vi "G# - InterfaceDemo2.vi"() -> ()   [LabVIEW 2017]
doc: "G# Interface Implementation\nThis examples demonstrates how to use the G#Interface. The interface concept is an alternative design principle to multiple inheritance (just as in C# and Java). Classes that are not related can implement the same interface and the reference of the interface could be treated just as they are from the same class.\n\nBy using the G# Debugger found in Tools->G# Debugger a text log can be followed showing how the objects were created and destroyed."
uses:
  IMyInterface2_interface/IMyInterface2.lvclass
  C:/ProjectGSharpDevelopment_2017/gsharp/VIPM/Files/vi.lib/addons/_AddQ/G#Object/G#Object.lvclass
  MyClass3_class/MyClass3.lvclass
  MyClass4_class/MyClass4.lvclass
  vi.lib/addons/_AddQ/G#Object/G#Object.lvclass
panel:
  out "# of objects killed":i32
  out "OK":bool
  in  "error in (no error)":errorcluster
  out "MyClass4 is instance of IMyInterface":bool
  out "MyClass3 is instance of IMyInterface":bool
  out "error out":errorcluster
  out "Class Name":string[](array[string])
  # "G# Interface Implementation without wrapper classes\nThis examples demonstrates how to use the G#Interface without using wrapper classes. The interface concept is an alternative design principle to multiple inheritance (just as in C# and Java).\nClasses that are not related can implement the same interface and the reference of the interface could be treated just as they are from the same class.\n\nBy using the G# Debugger found in Tools->G# Debugger a text log can be followed showing how the objects were created and destroyed."
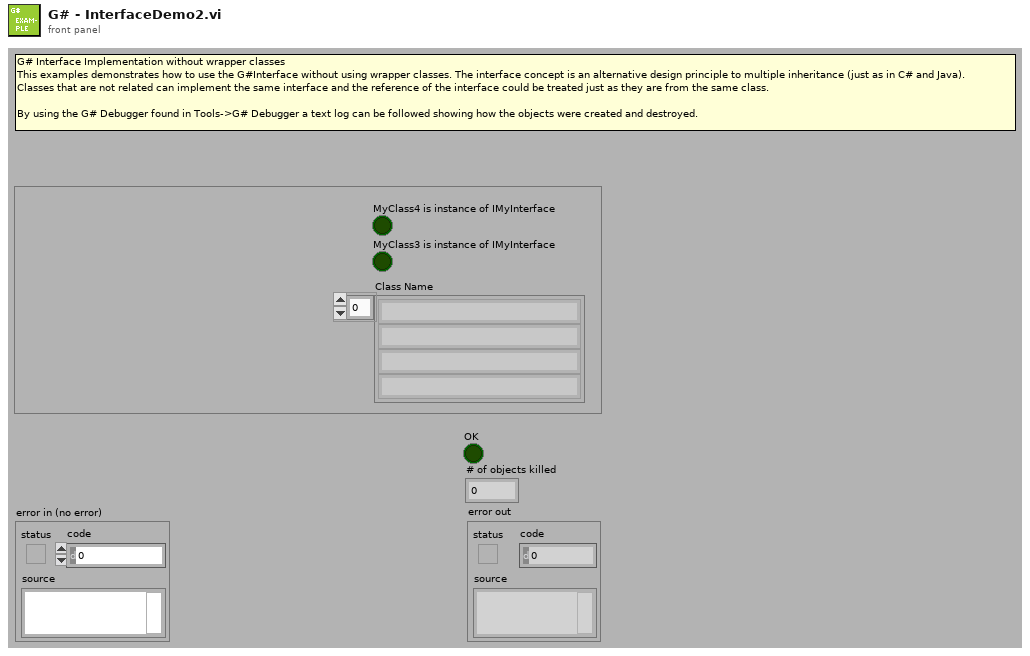
[diagram p1: front panel]
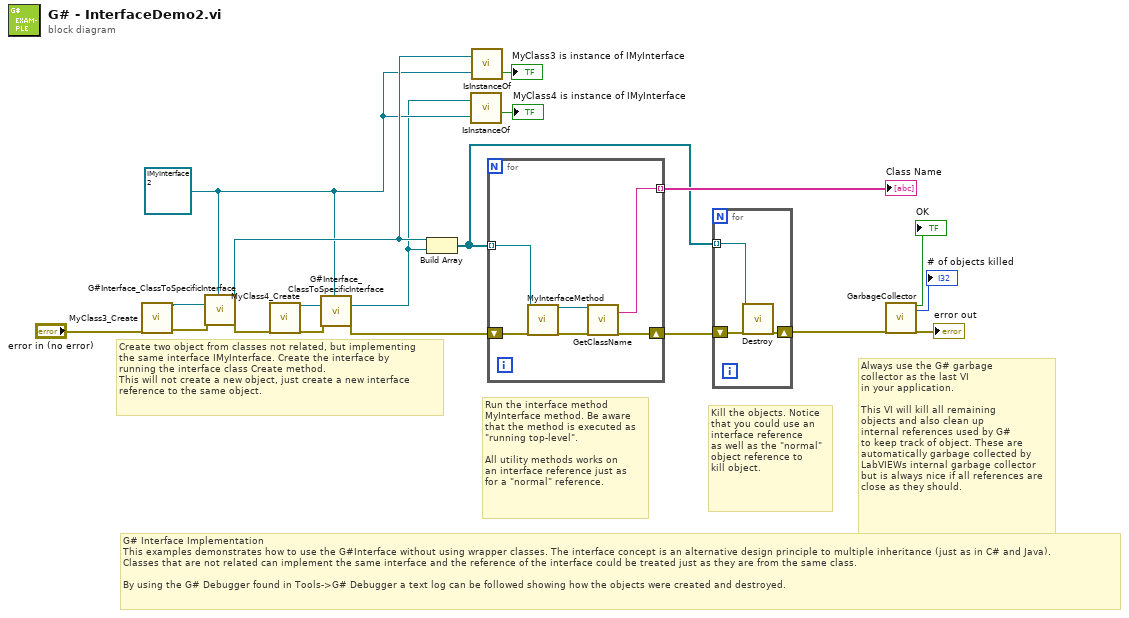
[diagram p0: block diagram]
diagram:
  w2 = refnum<class "IMyInterface2.lvclass"> refnum ("IMyInterface2.lvclass")
  # "G# Interface Implementation\nThis examples demonstrates how to use the G#Interface without using wrapper classes. The interface concept is an alternative design principle to multiple inheritance (just as in C# and Java).\nClasses that are not related can implement the same interface and the reference of the interface could be treated just as they are from the same class.\n\nBy using the G# Debugger found in Tools->G# Debugger a text log can be followed showing how the objects were created and destroyed."
  # "Always use the G# garbage\ncollector as the last VI\nin your application.\n\nThis VI will kill all remaining\nobjects and also clean up\ninternal references used by G#\nto keep track of object. These are\nautomatically garbage collected by\nLabVIEWs internal garbage collector\nbut is always nice if all references are\nclose as they should."
  # "Kill the objects. Notice\nthat you could use an\ninterface reference\nas well as the \"normal\"\nobject reference to\nkill object."
  # "Run the interface method\nMyInterface method. Be aware\nthat the method is executed as\n\"running top-level\".\n\nAll utility methods works on\nan interface reference just as\nfor a \"normal\" reference."
  # "Create two object from classes not related, but implementing\nthe same interface IMyInterface. Create the interface by\nrunning the interface class Create method.\nThis will not create a new object, just create a new interface\nreference to the same object."
  n1 = call "MyClass3_Create.vi"("error in (no error)"="error in (no error)") -> ("reference out"=w7:refnum<class "MyClass3.lvclass">, "error out"=w9:errorcluster)  [unwired: 17 in]
  n2 = call-dynamic "G#Interface_ClassToSpecificInterface.vi"("reference in"=w7, "error in (no error)"=w9, "target interface"=w2) -> ("interface reference out"=w6:refnum<class "IMyInterface2.lvclass">, "error out"=w8:errorcluster)  [unwired: 23 in]
  n3 = call "MyClass4_Create.vi"("error in (no error)"=w8) -> ("reference out"=w5:refnum<class "MyClass4.lvclass">, "error out"=w4:errorcluster)  [unwired: 17 in]
  n4 = call-dynamic "G#Interface_ClassToSpecificInterface.vi"("reference in"=w5, "error in (no error)"=w4, "target interface"=w2) -> ("interface reference out"=w1:refnum<class "IMyInterface2.lvclass">, "error out"=w3:errorcluster)  [unwired: 23 in]
  n5 = Build Array(w6, w1) -> (w15:refnum<class "IMyInterface2.lvclass">[])
  n6 = call-dynamic "IsInstanceOf.vi"("is object instance of"=w2, "reference in"=w1) -> ("is instance of"=→"MyClass4 is instance of IMyInterface":bool)  [unwired: 1 out]
  n7 = call-dynamic "IsInstanceOf.vi"("is object instance of"=w2, "reference in"=w6) -> ("is instance of"=→"MyClass3 is instance of IMyInterface":bool)  [unwired: 1 out]
  n8 = for {
    shift-right: [w22] -> w18
    shift-left: w3 -> [w25]
    tunnel: w15 -> [w24] mode=indexing
    tunnel: [w20] -> w17 mode=indexing
    n9 = call-dynamic "MyInterfaceMethod.vi"("reference in"=w24, "error in (no error)"=w25) -> ("reference out"=w21:refnum<class "IMyInterface2.lvclass">, "error out"=w23:errorcluster)  [unwired: 16 in]
    n10 = call-dynamic "GetClassName.vi"("reference in"=w21, "error in (no error)"=w23) -> ("class name"=w20:string, "error out"=w22:errorcluster)  [unwired: 13 in, 3 out]
  }
  "Class Name" <- w17
  n11 = for {
    shift-right: [w27] -> w16
    shift-left: w18 -> [w28]
    tunnel: w15 -> [w26] mode=indexing
    n12 = call-dynamic "Destroy.vi"("reference in"=w26, "error in (no error)"=w28) -> ("error out"=w27:errorcluster)  [unwired: 16 in, 1 out]
  }
  n13 = call "GarbageCollector.vi"("error in (no error)"=w16) -> ("OK"=→"OK":bool, "# of objects killed"=→"# of objects killed":i32, "error out"=→"error out":errorcluster)  [unwired: 16 in]
